vi "Initialize Scan Angle Data.vi"(6 "initial angle (0)":dbl, 9 "scan angle":dbl, 10 "min angle":dbl, 11 "max angle":dbl) -> (1 "scan angle used":dbl, 3 "scan angles":T1)   [LabVIEW 2017, in "NI_Robotics_Scan Angles.lvlib"]
uses:
  <vilib>/robotics/Utilities/Scan Angles/NI_Robotics_Scan Angles.lvlib
  <vilib>/robotics/Utilities/Scan Angles/Scan Angle Data.ctl
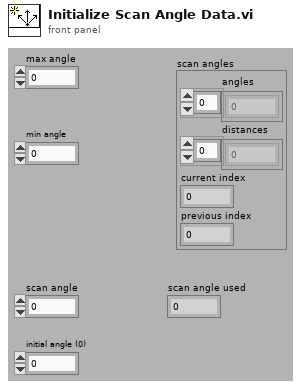
[diagram p1: front panel]
types:
  T1 = typedef "NI_Robotics_Scan Angles.lvlib/Scan Angle Data.ctl" = cluster{"angles":dbl[], "distances":dbl[], "current index":i32, "previous index":i32}
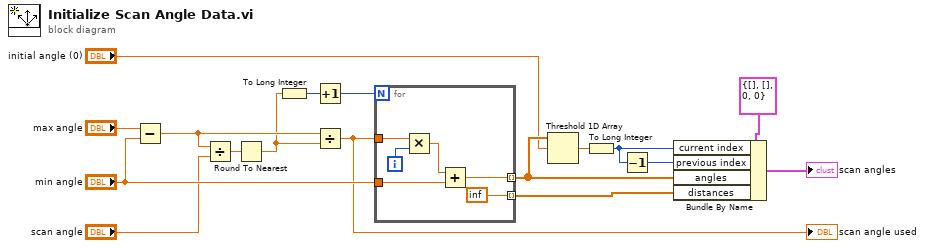
[diagram p0: block diagram]
diagram:
  n1 = Subtract(x="max angle", y="min angle") -> (x-y=w6:dbl)
  n2 = Divide(x=w6, y="scan angle") -> (x/y=w4:dbl)
  n3 = Round To Nearest(number=w4) -> (nearest integer value=w2:dbl)
  n4 = To Long Integer(number=w2) -> (32bit integer=w1:i32)
  n5 = Increment(x=w1) -> (x+1=w3:i32)
  n6 = Divide(x=w6, y=w2) -> (x/y=w12:dbl)
  "scan angle used" <- w12
  n7 = for {
    N: w3 -> [_]
    tunnel: "min angle" -> [w21]
    tunnel: w12 -> [w23]
    tunnel: [w19] -> w11 mode=indexing
    tunnel: [inf] -> w16 mode=indexing
    i -> [w22]
    n8 = Multiply(x=w23, y=w22) -> (x*y=w20:dbl)
    n9 = Add(x=w20, y=w21) -> (x+y=w19:dbl)
  }
  n10 = Threshold 1D Array(2:"initial angle (0)", 3:w11) -> (0:w9:dbl)  [unwired: 1 in]
  n11 = To Long Integer(number=w9) -> (32bit integer=w8:i32)
  n12 = Decrement(x=w8) -> (x-1=w7:i32)
  n13 = Bundle By Name(cluster=T1 {"angles"=[], "distances"=[], "current index"=0, "previous index"=0} ("obstacle vectors"), "current index"=w8, "previous index"=w7, "angles"=w11, "distances"=w16) -> (→"scan angles":T1)
